vi "5~15radom_numbers-4.21.vi"() -> ()   [LabVIEW 2015]
panel:
  in  "Stop Button":bool
  out "Waveform Chart":dbl(graph)
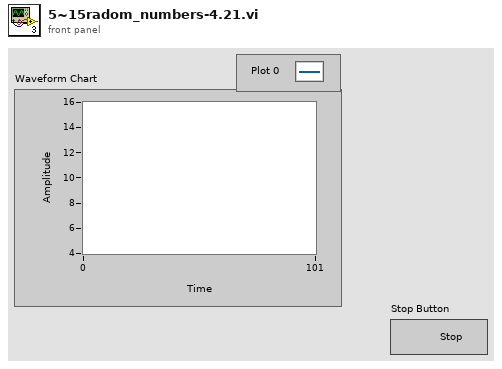
[diagram p1: front panel]
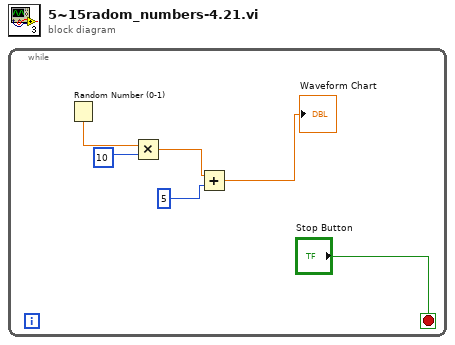
[diagram p0: block diagram]
diagram:
  n1 = while {
    stop <- "Stop Button" stop-if-true
    n2 = Random Number (0-1)() -> (number: 0 to 1=w4:dbl)
    n3 = Multiply(x=w4, y=10) -> (x*y=w3:dbl)
    n4 = Add(x=w3, y=5) -> (x+y=→"Waveform Chart":dbl)
  }
